vi "Read Trace.vi"(8 "error in (no error)":errorcluster, 10 "Resolution (0: High Resolution)":i32(ring) items=["High Resolution", "Medium Resolution", "Low Resolution"], 11 "VISA resource name":refnum<visa-resource-name>) -> (0 "error out":errorcluster, 2 "Trace Data":dbl[](array[numeric]), 3 "VISA resource name out":refnum<visa-resource-name>)   [LabVIEW 2018, in "Agilent U2000 Series.lvlib"]
doc: "Returns trace data with the specified resolution.\n\nNote:\n(1) Only available when trace is enabled by <b>Configure Trace.vi</b>\n(2) Not available for U2004A model\n(3) In case of U2040 X-Series, it is applicable for U2042XA/U2044XA/U2049XA only."
uses:
  Agilent U2000 Series.lvlib
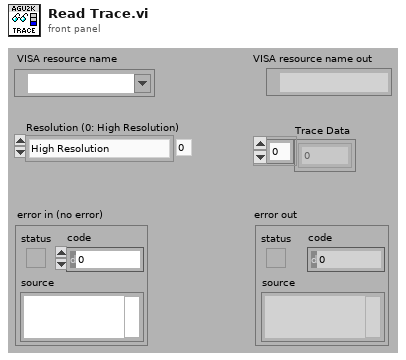
[diagram p1: front panel]
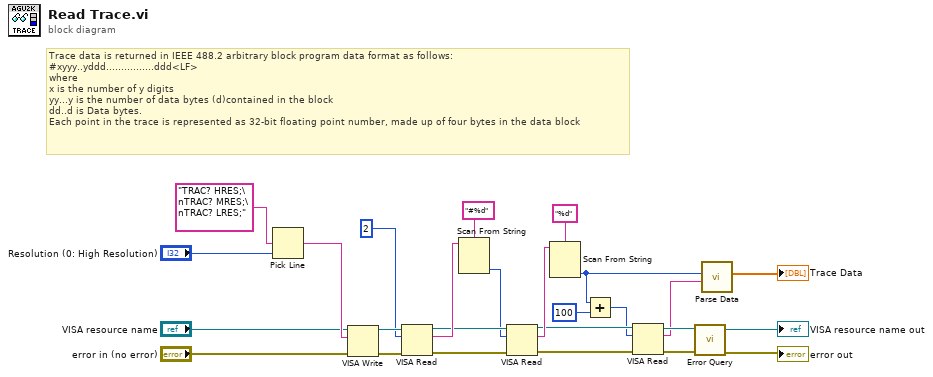
[diagram p0: block diagram]
diagram:
  # "Trace data is returned in IEEE 488.2 arbitrary block program data format as follows:\n#xyyy..yddd................ddd<LF>\nwhere \nx is the number of y digits\nyy...y is the number of data bytes (d)contained in the block\ndd..d is Data bytes. \nEach point in the trace is represented as 32-bit floating point number, made up of four bytes in the data block"
  n1 = Pick Line(multi-line string="TRAC? HRES;\nTRAC? MRES;\nTRAC? LRES;", line index="Resolution (0: High Resolution)") -> (output string=w24:string)  [unwired: 1 out]
  n2 = VISA Write(VISA resource name="VISA resource name", write buffer=w24, error in (no error)="error in (no error)") -> (VISA resource name out=w20:refnum<visa-resource-name>, error out=w21:errorcluster)  [unwired: 1 out]
  n3 = VISA Read(VISA resource name=w20, byte count=u32 2, error in (no error)=w21) -> (VISA resource name out=w16:refnum<visa-resource-name>, read buffer=w18:string, error out=w15:errorcluster)  [unwired: 1 out]
  n4 = Scan From String(format string="#%d", input string=w18) -> (output 1=w14:i32)  [unwired: 2 in, 4 out]
  n5 = VISA Read(VISA resource name=w16, byte count=w14, error in (no error)=w15) -> (VISA resource name out=w11:refnum<visa-resource-name>, read buffer=w12:string, error out=w10:errorcluster)  [unwired: 1 out]
  n6 = Scan From String(format string="%d", input string=w12) -> (output 1=w3:i32)  [unwired: 2 in, 4 out]
  n7 = Add(x=w3, y=100) -> (x+y=w8:i32)
  n8 = VISA Read(VISA resource name=w11, byte count=w8, error in (no error)=w10) -> (VISA resource name out=w7:refnum<visa-resource-name>, read buffer=w2:string, error out=w6:errorcluster)  [unwired: 1 out]
  n9 = call "Error Query.vi"("error in (no error)"=w6, "VISA resource name"=w7) -> ("error out"=→"error out":errorcluster, "VISA resource name out"=→"VISA resource name out":refnum<visa-resource-name>)  [unwired: 8 out]
  n10 = call "Parse Data.vi"("Read Buffer"=w2, "Data Length"=w3) -> ("Output Data Array"=→"Trace Data":dbl[])  [unwired: 9 out]
